vi "Notifier.vi"() -> ()   [LabVIEW 2021]
panel:
  out "Consumer Loop":dbl(graph)
  out "Producer Loop":dbl(graph)
  in  "stop":bool
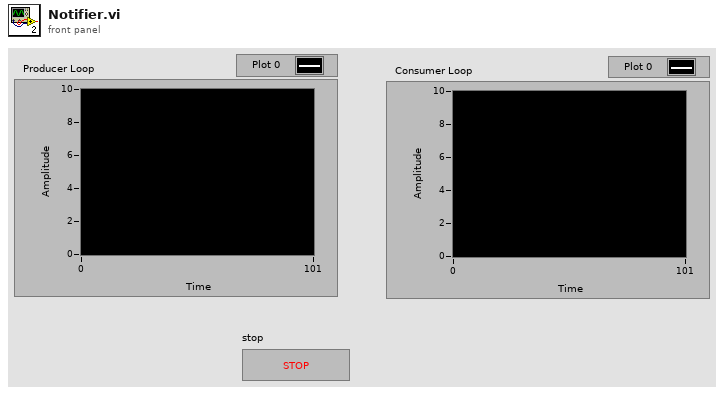
[diagram p1: front panel]
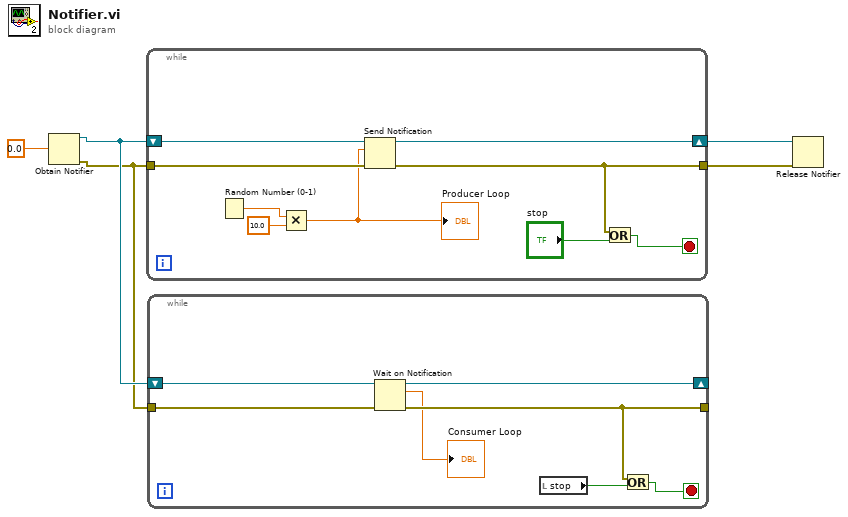
[diagram p0: block diagram]
diagram:
  n1 = Obtain Notifier(notification data type=0.0) -> (notifier out=w2:refnum<notifier>, error out=w1:errorcluster)  [unwired: 3 in, 1 out]
  n2 = while {
    tunnel: w1 -> [w13]
    tunnel: [w11] -> w4
    shift-right: [w12] -> w5
    shift-left: w2 -> [w14]
    stop <- w10 stop-if-true
    n3 = Random Number (0-1)() -> (number: 0 to 1=w8:dbl)
    n4 = Multiply(x=w8, y=10.0) -> (x*y=w6:dbl)
    "Producer Loop" <- w6
    n5 = Send Notification(notification=w6, notifier=w14, error in (no error)=w13) -> (notifier out=w12:refnum<notifier>, error out=w11:errorcluster)
    n6 = Or(x=w11, y="stop") -> (x .or. y?=w10:bool)
  }
  n7 = while {
    tunnel: w1 -> [w20]
    tunnel: [w16] -> _
    shift-right: [w17] -> _
    shift-left: w2 -> [w21]
    stop <- w18 stop-if-true
    n8 = Wait on Notification(notifier=w21, error in (no error)=w20) -> (notifier out=w17:refnum<notifier>, notification=→"Consumer Loop":dbl, error out=w16:errorcluster)  [unwired: 2 in, 1 out]
    n9 = local read "stop"() -> (w19:bool)
    n10 = Or(x=w16, y=w19) -> (x .or. y?=w18:bool)
  }
  n11 = Release Notifier(notifier=w5, error in (no error)=w4) -> ()  [unwired: 1 in, 3 out]
